vi "Prepare Delete Row Command.vi"(8 "Error In (no error)":errorcluster, 10 "Record":variant) -> (0 "Error Out":errorcluster, 2 "Insert SQL Command":string)   [LabVIEW 2023, in "SQLite DB Operator.lvclass"]
uses:
  SQLite DB Operator.lvclass
  SQLite DB Operator.lvclass/SQLite DB Operator.ctl
  <vilib>/Utility/Data Type/NI_Data Type.lvlib
  <userlib>/_OpenG.lib/array/array.llb/Delete Elements from 1D Array (String)__ogtk.vi
  <userlib>/_OpenG.lib/array/array.llb/Search 1D Array (String)__ogtk.vi
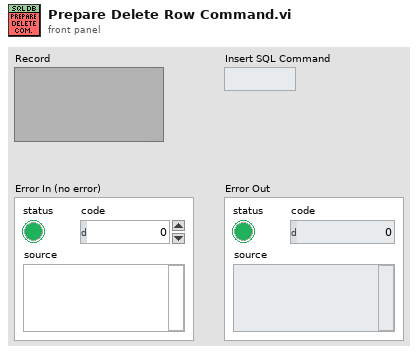
[diagram p1: front panel]
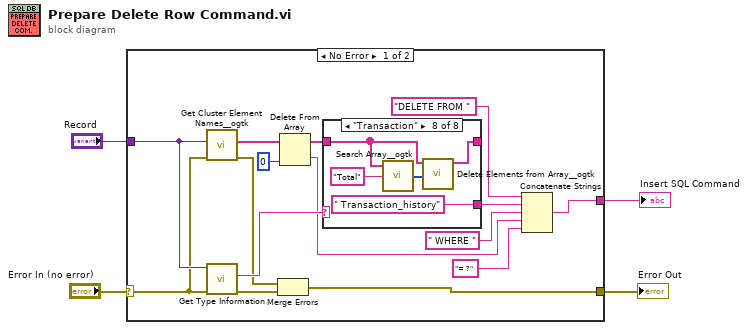
[diagram p0: block diagram]
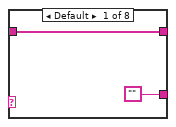
[diagram p2: hidden frame]
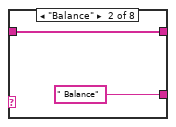
[diagram p3: hidden frame]
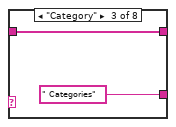
[diagram p4: hidden frame]
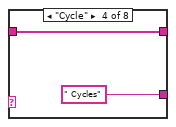
[diagram p5: hidden frame]
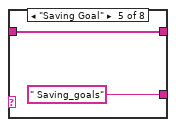
[diagram p6: hidden frame]
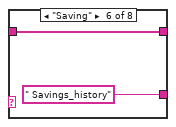
[diagram p7: hidden frame]
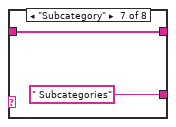
[diagram p8: hidden frame]
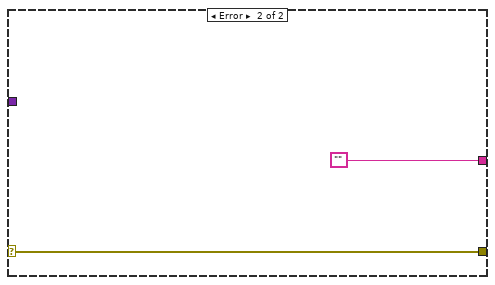
[diagram p9: hidden frame]
diagram:
  n1 = case shown="No Error" "Error In (no error)" {
    selector: "Error In (no error)" -> [w10 w40]
    tunnel: [w17 w40] -> w4
    tunnel: [w8 ""] -> w3
    tunnel: "Record" -> [w11 _]
    frame No Error {
      n2 = call <userlib>:"Get Cluster Element Names__ogtk.vi"("error in (no error)"=w10, "Cluster"=w11) -> ("error out"=w14:errorcluster, "Element Names"=w13:string[])  [unwired: 8 in]
      n3 = call <vilib>:"Get Type Information.vi"("error in (no error)"=w10, "variant"=w11) -> ("error out"=w15:errorcluster, "name"=w19:string)  [unwired: 5 in, 3 out]
      n4 = Merge Errors(w14, w15) -> (w17:errorcluster)
      n5 = Delete From Array(array=w13, index=0) -> (deleted portion=w6:string, array with subset deleted=w9:string[])  [unwired: 1 in]
      n6 = case shown="\"Transaction\"" w19 {
        tunnel: ["" " Balance" ("string") " Categories" ("string") " Cycles" ("string") " Saving_goals" ("string") " Savings_history" ("string") " Subcategories" ("string") " Transaction_history" ("string")] -> w16
        tunnel: w9 -> [w20 w22 w24 w26 w28 w30 w32 w35]
        tunnel: [w20 w22 w24 w26 w28 w30 w32 w34] -> _
        frame Default {
        }
        frame "Balance" {
        }
        frame "Category" {
        }
        frame "Cycle" {
        }
        frame "Saving Goal" {
        }
        frame "Saving" {
        }
        frame "Subcategory" {
        }
        frame "Transaction" {
          n7 = call-poly <userlib>:"Search Array__ogtk.vi"("Array"=w35, "Element Data"="Total") -> ("Indices of Elements"=w36:i32[])  [unwired: 7 in]
          n8 = call-poly <userlib>:"Delete Elements from Array__ogtk.vi"("indices"=w36, "array"=w35) -> ("array w/ subset deleted"=w34:string[])  [unwired: 8 in, 1 out]
        }
      }
      n9 = Concatenate Strings("DELETE FROM ", w16, " WHERE ", w6, "= ?") -> (w8:string)
    }
    frame Error {
    }
  }
  "Error Out" <- w4
  "Insert SQL Command" <- w3
